vi "Configure Feed Forward Equalization.vi"(0 "VISA resource name":refnum<visa-resource-name>, 1 "Bandwidth Mode (0: Track Scope Bandwidth)":i32(ring) items=["Track Scope Bandwidth", "Track Tap Delay", "Custom"], 2 "Bandwidth (4 GHz)":dbl=4000000000.0, 5 "Enable FFE (T: Enable)":bool=TRUE, 7 "FFE Source (1: Channel 1)":i32(ring)=1 items=["Channel 1"=1, "Channel 2"=2, "Channel 3"=3, "Channel 4"=4, "Function 1"=5, "Function 2"=6, "Function 3"=7, "Function 4"=8, "Memory 1"=9, "Memory 2"=10, "Memory 3"=11, "Memory 4"=12, "Differential 1"=13, "Differential 2"=14, "Common 1"=15, "Common 2"=16], 9 "Drift (1 ms)":dbl=0.001, 11 "error in (no error)":errorcluster, 12 "Delay Mode (0: Track Date Rate)":i32(ring) items=["Track Data Rate", "Custom"], 13 "Delay (400 ps)":dbl=4e-10) -> (4 "VISA resource name out":refnum<visa-resource-name>, 15 "error out":errorcluster)   [LabVIEW 2020, in "Agilent 90000 Series.lvlib"]
doc: "Configures the basic settings for Decision Feedback Equalization."
uses:
  Agilent 90000 Series.lvlib
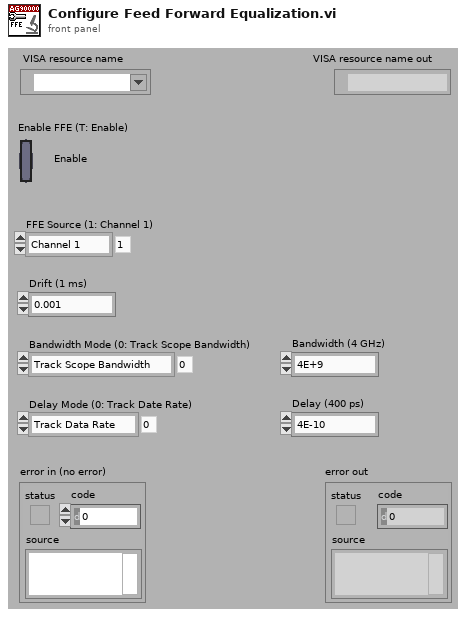
[diagram p1: front panel]
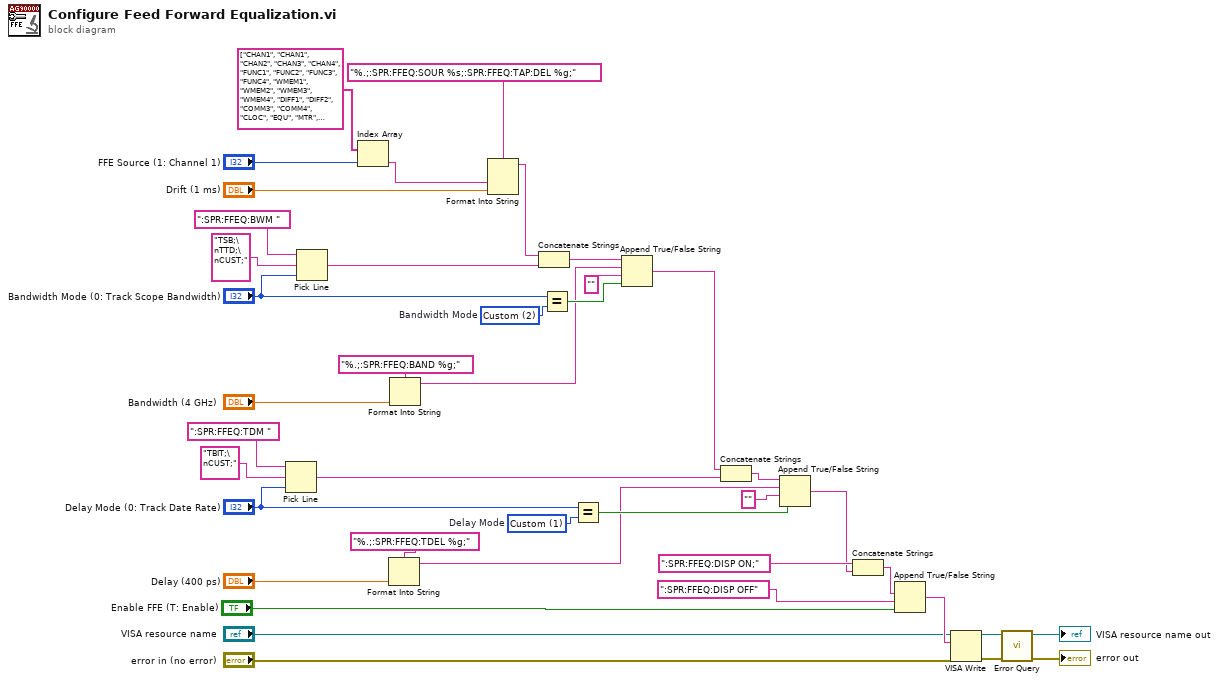
[diagram p0: block diagram]
diagram:
  w14 = 1 items=["Track Data Rate", "Custom"]  # Delay Mode
  w21 = 2 items=["Track Scope Bandwidth", "Track Tap Delay", "Custom"]  # Bandwidth Mode
  n1 = Pick Line(string ("")=":SPR:FFEQ:TDM ", multi-line string="TBIT;\nCUST;", line index="Delay Mode (0: Track Date Rate)") -> (output string=w15:string)
  n2 = Pick Line(string ("")=":SPR:FFEQ:BWM ", multi-line string="TSB;\nTTD;\nCUST;", line index="Bandwidth Mode (0: Track Scope Bandwidth)") -> (output string=w23:string)
  n3 = Index Array(array=string[] ["CHAN1", "CHAN1", "CHAN2", "CHAN3", "CHAN4", "FUNC1", "FUNC2", "FUNC3", "FUNC4", "WMEM1", "WMEM2", "WMEM3", "WMEM4", "DIFF1", "DIFF2", "COMM3", "COMM4", "CLOC", "EQU", "MTR", "MSP"] ("subarray 2"), index="FFE Source (1: Channel 1)") -> (element=w32:string)
  n4 = Format Into String(format string="%.;:SPR:FFEQ:TDEL %g;", "Delay (400 ps)") -> (resulting string=w11:string)  [unwired: 2 in, 1 out]
  n5 = Format Into String(format string="%.;:SPR:FFEQ:BAND %g;", "Bandwidth (4 GHz)") -> (resulting string=w19:string)  [unwired: 2 in, 1 out]
  n6 = Format Into String(format string="%.;:SPR:FFEQ:SOUR %s;:SPR:FFEQ:TAP:DEL %g;", w32, "Drift (1 ms)") -> (resulting string=w24:string)  [unwired: 2 in, 1 out]
  n7 = Concatenate Strings(w24, w23) -> (w17:string)
  n8 = Equal?(x="Bandwidth Mode (0: Track Scope Bandwidth)", y=w21) -> (x = y?=w22:bool)
  n9 = Equal?(x="Delay Mode (0: Track Date Rate)", y=w14) -> (x = y?=w12:bool)
  n10 = Append True/False String(1:w22, 2:"" ("false string"), 3:w19, 4:w17) -> (0:w16:string)
  n11 = Concatenate Strings(w16, w15) -> (w9:string)
  n12 = Append True/False String(1:w12, 2:"" ("false string"), 3:w11, 4:w9) -> (0:w6:string)
  n13 = Concatenate Strings(":SPR:FFEQ:DISP ON;" ("false string"), w6) -> (w5:string)
  n14 = Append True/False String(1:"Enable FFE (T: Enable)", 2:":SPR:FFEQ:DISP OFF" ("false string"), 3:w5) -> (0:w3:string)  [unwired: 1 out]
  n15 = VISA Write(VISA resource name="VISA resource name", write buffer=w3, error in (no error)="error in (no error)") -> (VISA resource name out=w39:refnum<visa-resource-name>, error out=w38:errorcluster)  [unwired: 1 out]
  n16 = call "Error Query.vi"("error in (no error)"=w38, "VISA resource name"=w39) -> ("error out"=→"error out":errorcluster, "VISA resource name out"=→"VISA resource name out":refnum<visa-resource-name>)  [unwired: 8 out]
